vi "Periodic Tasks.vi"(8 "error in":errorcluster) -> ()   [LabVIEW 2014]
doc: "This VI runs in parallel to other tasks. It can contain as many user-defined periodic loops as you need. These can carry out PID or other sorts of timed response."
uses:
  <vilib>/Rock Robotics/SystemInterfaces/Utilities/FPGA_UtilitiesLED Source.ctl
  <vilib>/Rock Robotics/SystemInterfaces/Utilities/FPGA_UtilitiesLED State.ctl
  <vilib>/Rock Robotics/WPI/Joystick/WPI_JoystickGetSetRefNum.vi
  <vilib>/Rock Robotics/WPI/RobotDrive/WPI_RobotDriveGetSetRefNum.vi
  <vilib>/Rock Robotics/Network Tables/SD Write Number.vi
  <vilib>/Rock Robotics/Network Tables/SD Write Boolean.vi
  Global 1.vi
  Robot Global Data.vi
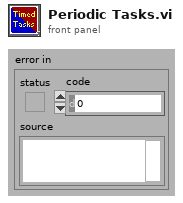
[diagram p1: front panel]
types:
  T1 = typedef "WPI_JoystickDevRef.ctl" = cluster{"Device":T2}
  T2 = typedef "WPI_JoystickDeviceEnum.ctl" = enum16{"USB 0", "USB 1", "USB 2", "USB 3", "USB 4", "USB 5"}
  T3 = typedef "WPI_RobotDriveDevRef.ctl" = cluster{"DevStatus":errorcluster, "Motors[]":T4[], "Square Inputs":bool, "Max Output":dbl}
  T4 = typedef "WPI_MotorControlDeviceRef.ctl" = cluster{"DeviceStatus":errorcluster, "Type":enum16{"PWM", "CAN"}, "PWM":cluster{"Digital Module":T5, "PWM Channel":T6, "DeadBand":T7}, "CAN":cluster{"Device Number":u8, "Control Mode":T8, "Semaphore":T9, "Max Vout":dbl}, "Invert":bool, "TransformRef":T10, "InvTransformRef":T10}
  T5 = typedef "FPGA_TypedefDigitalModule.ctl" = enum16{"Digital Module 1", "Digital Module 2"}
  T6 = typedef "FPGA_DIOPWMChannel.ctl" = enum8{"PWM 1", "PWM 2", "PWM 3", "PWM 4", "PWM 5", "PWM 6", "PWM 7", "PWM 8", "PWM 9", "PWM 10", "Invalid"}
  T7 = typedef "WPI_PWMDeadband.ctl" = cluster{"Name":string, "maxPositivePwm":i32, "minPositivePwm":i32, "centerPwm":i32, "maxNegativePwm":i32, "minNegativePwm":i32, "angularRange":u16}
  T8 = typedef "WPI_CANJaguar_ControlMode.ctl" = enum8{"Percent VBus", "Current", "Speed", "Position", "Voltage"}
  T9 = typedef "Semaphore RefNum" = refnum<k1>
  T10 = typedef "WPI_PWMTransform_ConPane.ctl" = refnum<vi>
  T11 = cluster{"JoystickDevRef":T1, "RobotDriveDevRef":T3}
  T12 = typedef "WPI_EncoderDevRef.ctl" = cluster{"DevStatus":errorcluster, "EncoderIndex":T13, "CounterIndex":T14, "DistancePerCount":dbl, "Decoding Type":T15}
  T13 = typedef "FPGA_EncoderIdx.ctl" = enum8{"Enc 0", "Enc 1", "Enc 2", "Enc 3", "Invalid"}
  T14 = typedef "FPGA_CounterCtrSystemIndex.ctl" = enum8{"Ctr 0", "Ctr 1", "Ctr 2", "Ctr 3", "Ctr 4", "Ctr 5", "Ctr 6", "Ctr 7", "Invalid"}
  T15 = typedef "WPI_EncoderType.ctl" = enum16{"1x", "2x", "4x"}
  T16 = typedef "FPGA_UtilitiesLED State.ctl" = enum16{"Off", "On", "Toggle"}
  T17 = typedef "FPGA_UtilitiesLED Source.ctl" = enum16{"User LED", "FPGA LED"}
  T18 = typedef "WPI_CompressorDevRef.ctl" = cluster{"DevStatus":errorcluster, "DigitalInputDevRef":T19, "RelayDevRef":T21}
  T19 = typedef "WPI_DigitalInputDevRef.ctl" = cluster{"DevStatus":errorcluster, "DIO Channel":T20, "Digital Module":T5}
  T20 = typedef "FPGA_DIOChannel.ctl" = enum8{"DIO 1", "DIO 2", "DIO 3", "DIO 4", "DIO 5", "DIO 6", "DIO 7", "DIO 8", "DIO 9", "DIO 10", "DIO 11", "DIO 12", "DIO 13", "DIO 14", "Invalid"}
  T21 = typedef "WPI_RelayDevRef.ctl" = cluster{"DevStatus":errorcluster, "Relay Channel":T22, "Digital Module":T5, "Relay Direction":T23}
  T22 = typedef "FPGA_DIORelayChannel.ctl" = enum8{"Relay 1", "Relay 2", "Relay 3", "Relay 4", "Relay 5", "Relay 6", "Relay 7", "Relay 8", "Invalid"}
  T23 = typedef "WPI_RelayDirection.ctl" = enum16{"Both directions", "Forward only", "Reverse only"}
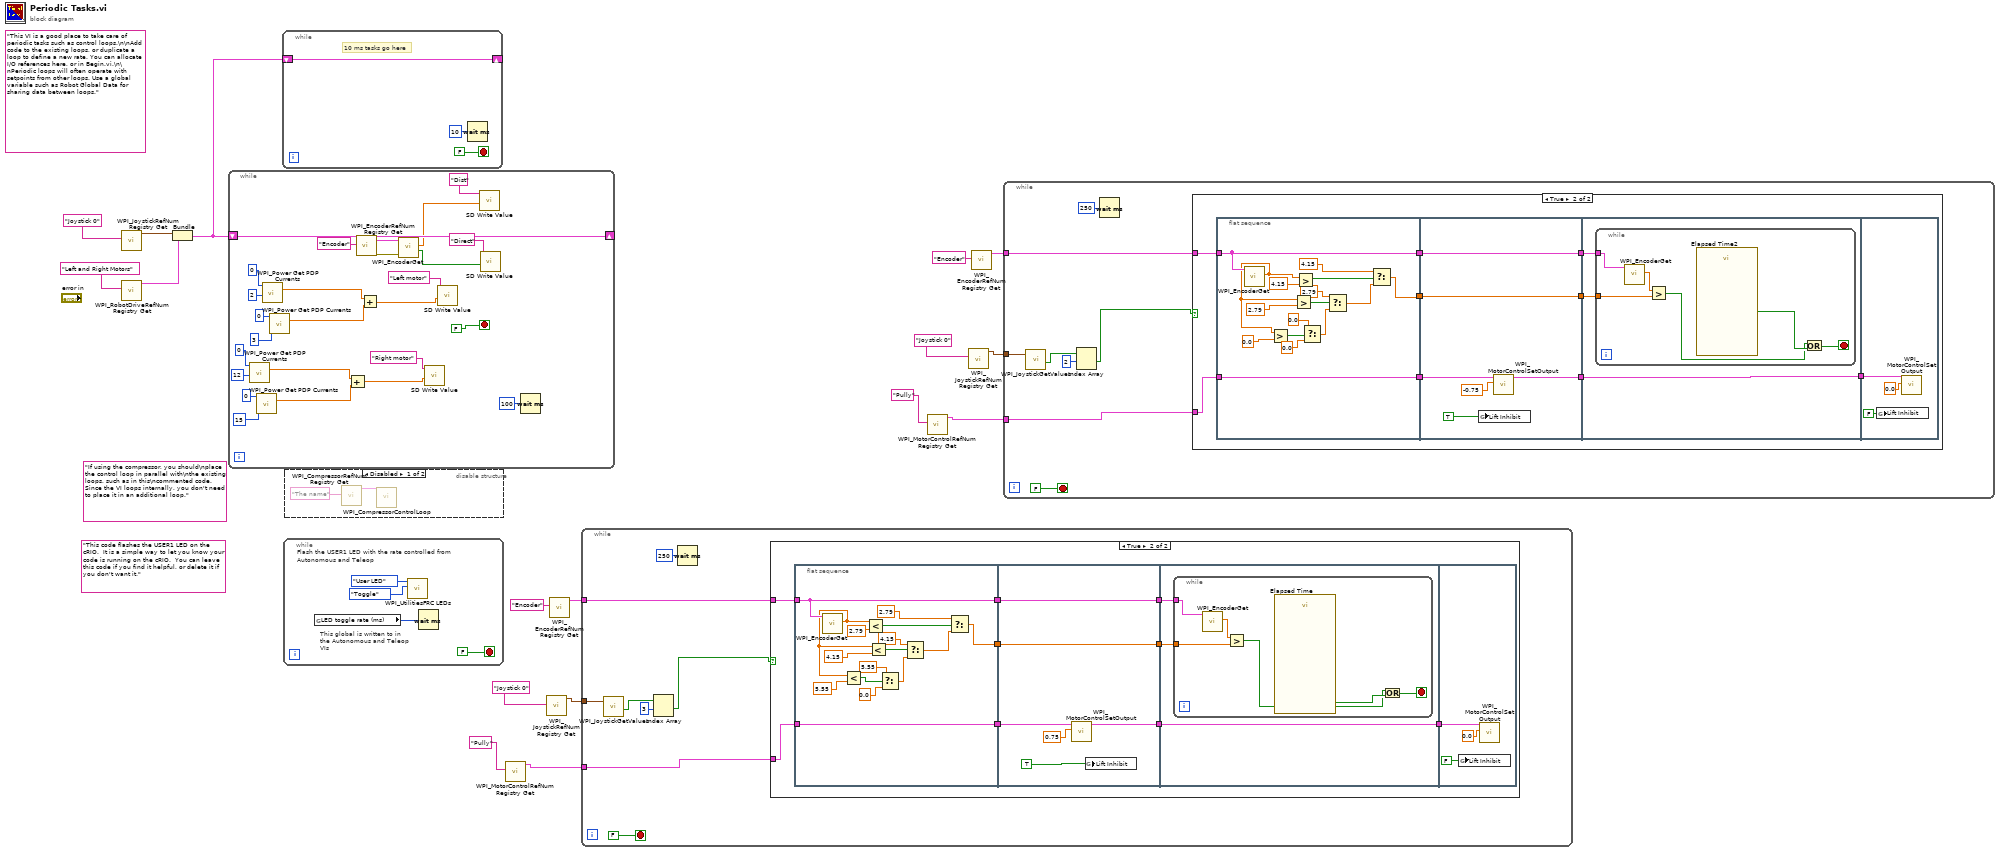
[diagram p0: block diagram]
diagram:
  (unwired) "If using the compressor, you should\nplace the control loop in parallel with\nthe existing loops, such as in this\ncommented code. Since the VI loops internally, you don't need to place it in an additional loop."
  (unwired) "This code flashes the USER1 LED on the cRIO.  It is a simple way to let you know your code is running on the cRIO.  You can leave this code if you find it helpful, or delete it if you don't want it."
  (unwired) "This VI is a good place to take care of periodic tasks such as control loops.\n\nAdd code to the existing loops, or duplicate a loop to define a new rate. You can allocate I/O references here, or in Begin.vi.\n\nPeriodic loops will often operate with setpoints from other loops. Use a global variable such as Robot Global Data for sharing data between loops."
  n1 = call <vilib>:"WPI_JoystickRefNum Registry Get.vi"("refnum name"="Joystick 0") -> ("JoystickDevRef"=w15:T1)  [unwired: 1 in, 9 out]
  n2 = call <vilib>:"WPI_RobotDriveRefNum Registry Get.vi"("refnum name"="Left and Right Motors") -> ("RobotDriveDevRef"=w14:T3)  [unwired: 1 in, 9 out]
  n3 = Bundle("JoystickDevRef"=w15, "RobotDriveDevRef"=w14) -> (w13:T11)  [unwired: 1 out]
  n4 = while {
    shift-right: [w43] -> _
    shift-left: w13 -> [w43]
    stop <- FALSE stop-if-true
    n5 = call <vilib>:"WPI_Power Get PDP Currents.vi"("Power Distribution Panel (0)"=u8 0, "PDP Channel"=12) -> ("current (A)"=w29:dbl)  [unwired: 11 in, 2 out]
    n6 = call <vilib>:"WPI_Power Get PDP Currents.vi"("Power Distribution Panel (0)"=u8 0, "PDP Channel"=15) -> ("current (A)"=w28:dbl)  [unwired: 11 in, 2 out]
    n7 = call <vilib>:"WPI_Power Get PDP Currents.vi"("Power Distribution Panel (0)"=u8 0, "PDP Channel"=2) -> ("current (A)"=w37:dbl)  [unwired: 11 in, 2 out]
    n8 = call <vilib>:"WPI_Power Get PDP Currents.vi"("Power Distribution Panel (0)"=u8 0, "PDP Channel"=3) -> ("current (A)"=w36:dbl)  [unwired: 11 in, 2 out]
    n9 = Add(x=w29, y=w28) -> (x+y=w27:dbl)
    n10 = call <vilib>:"WPI_EncoderRefNum Registry Get.vi"("refnum name"="Encoder") -> ("error out"=w21:errorcluster, "EncoderDevRef"=w20:T12)  [unwired: 9 in]
    n11 = Add(x=w37, y=w36) -> (x+y=w35:dbl)
    n12 = call <vilib>:"WPI_EncoderGet.vi"("error in (no error)"=w21, "EncoderDevRef"=w20) -> ("Direction"=w24:bool, "Distance"=w22:dbl)  [unwired: 4 in, 4 out]
    n13 = call-poly <vilib>:"SD Write Value.vi"("Numeric"=w27, "Name"="Right motor") -> ()  [unwired: 8 in, 2 out]
    n14 = call-poly <vilib>:"SD Write Value.vi"("Numeric"=w35, "Name"="Left motor") -> ()  [unwired: 8 in, 2 out]
    n15 = call-poly <vilib>:"SD Write Value.vi"("Numeric"=w22, "Name"="Dist") -> ()  [unwired: 8 in, 2 out]
    n16 = call-poly <vilib>:"SD Write Value.vi"("Boolean"=w24, "Name"="Direct") -> ()  [unwired: 8 in, 2 out]
    n17 = Wait (ms)(milliseconds to wait=u32 100) -> ()  [unwired: 1 out]
  }
  n18 = while {
    shift-right: [w44] -> _
    shift-left: w13 -> [w44]
    stop <- FALSE stop-if-true
    # "10 ms tasks go here"
    n19 = Wait (ms)(milliseconds to wait=u32 10) -> ()  [unwired: 1 out]
  }
  n20 = while {
    stop <- FALSE stop-if-true
    # "This global is written to in the Autonomous and Teleop VIs"
    # "Flash the USER1 LED with the rate controlled from Autonomous and Teleop"
    n21 = global read "Robot Global Data.vi" "LED toggle rate (ms)"() -> (w47:u32)
    n22 = call <vilib>:"WPI_UtilitiesFRC LEDs.vi"("State"=FPGA_UtilitiesLED_State."Toggle", "LED Type"=FPGA_UtilitiesLED_Source."User LED") -> ()  [unwired: 1 in, 9 out]
    n23 = Wait (ms)(milliseconds to wait=w47) -> ()  [unwired: 1 out]
  }
  n24 = disable-structure shown="Disabled" {
    frame Disabled {
      n25 = call <vilib>:"WPI_CompressorRefNum Registry Get.vi"("refnum name"="The name") -> ("CompressorDevRef"=w52:T18)  [unwired: 9 in, 1 out]
      n26 = call <vilib>:"WPI_CompressorControlLoop.vi"("CompressorDevRef"=w52) -> ()  [unwired: 11 in]
    }
    frame Enabled {
    }
  }
  n27 = call <vilib>:"WPI_MotorControlRefNum Registry Get.vi"("refnum name"="Pully") -> ("MotorControlDevRef"=w11:T4)  [unwired: 9 in, 1 out]
  n28 = call <vilib>:"WPI_JoystickRefNum Registry Get.vi"("refnum name"="Joystick 0") -> ("JoystickDevRef"=w9:T1)  [unwired: 9 in, 1 out]
  n29 = call <vilib>:"WPI_EncoderRefNum Registry Get.vi"("refnum name"="Encoder") -> ("EncoderDevRef"=w8:T12)  [unwired: 9 in, 1 out]
  n30 = while {
    tunnel: w11 -> [w59]
    tunnel: w9 -> [w57]
    tunnel: w8 -> [w54]
    stop <- FALSE stop-if-true
    n31 = call <vilib>:"WPI_JoystickGetValues.vi"("JoystickDevRef"=w57) -> ("Buttons"=w56:bool[])  [unwired: 6 in, 4 out]
    n32 = Index Array(array=w56, index #1=3 ("index")) -> (element #1=w53:bool)  [unwired: 1 in, 1 out]
    n33 = Wait (ms)(milliseconds to wait=u32 250) -> ()  [unwired: 1 out]
    n34 = case shown="True" w53 {
      tunnel: w59 -> [_ w67]
      tunnel: w54 -> [_ w66]
      frame False {
      }
      frame True {
        n35 = flat-sequence {
          tunnel: w66 -> [w84]
          tunnel: w67 -> [w85]
          tunnel: [w85] -> w64
          tunnel: [w84] -> w63
          tunnel: [w70] -> w61
          tunnel: [w90] -> w69
          tunnel: [w88] -> w65
          tunnel: w64 -> [w91]
          tunnel: w63 -> [w88]
          tunnel: [w87] -> w62
          tunnel: w61 -> [w87]
          tunnel: w69 -> [w94]
          tunnel: [w94] -> w68
          tunnel: w65 -> [w93]
          tunnel: w62 -> [w92]
          tunnel: w68 -> [w103]
          frame #0 {
            n36 = call <vilib>:"WPI_EncoderGet.vi"("EncoderDevRef"=w84) -> ("Distance"=w79:dbl)  [unwired: 5 in, 5 out]
            n37 = Less?(x=w79, y=5.55) -> (x < y?=w74:bool)
            n38 = Less?(x=w79, y=2.79) -> (x < y?=w82:bool)
            n39 = Less?(x=w79, y=4.15) -> (x < y?=w75:bool)
            n40 = Select(t=5.55, s=w74, f=0.0) -> (s? t:f=w76:dbl)
            n41 = Select(t=4.15, s=w75, f=w76) -> (s? t:f=w77:dbl)
            n42 = Select(t=2.79, s=w82, f=w77) -> (s? t:f=w70:dbl)
          }
          frame #1 {
            n43 = call <vilib>:"WPI_MotorControlSetOutput.vi"("Output"=0.75, "MotorControlDevRef"=w91) -> ("MotorControlDevRef"=w90:T4)  [unwired: 7 in, 2 out]
            n44 = global write "Global 1.vi" "Lift Inhibit"(TRUE ("Lift Inhibit")) -> ()
          }
          frame #2 {
            n45 = while {
              tunnel: w93 -> [w97]
              tunnel: w92 -> [w95]
              stop <- w99 stop-if-true
              n46 = call <vilib>:"WPI_EncoderGet.vi"("EncoderDevRef"=w97) -> ("Distance"=w98:dbl)  [unwired: 5 in, 5 out]
              n47 = Greater?(x=w98, y=w95) -> (0:w96:bool)
              n48 = call "Elapsed Time"() -> ("Time has Elapsed"=w100:bool)  [unwired: 12 in, 7 out]
              n49 = Or(x=w96, y=w100) -> (x .or. y?=w99:bool)
            }
          }
          frame #3 {
            n50 = global write "Global 1.vi" "Lift Inhibit"(FALSE ("Lift Inhibit")) -> ()
            n51 = call <vilib>:"WPI_MotorControlSetOutput.vi"("Output"=0.0, "MotorControlDevRef"=w103) -> ()  [unwired: 7 in, 3 out]
          }
        }
      }
    }
  }
  n52 = call <vilib>:"WPI_MotorControlRefNum Registry Get.vi"("refnum name"="Pully") -> ("MotorControlDevRef"=w5:T4)  [unwired: 9 in, 1 out]
  n53 = call <vilib>:"WPI_JoystickRefNum Registry Get.vi"("refnum name"="Joystick 0") -> ("JoystickDevRef"=w3:T1)  [unwired: 9 in, 1 out]
  n54 = call <vilib>:"WPI_EncoderRefNum Registry Get.vi"("refnum name"="Encoder") -> ("EncoderDevRef"=w2:T12)  [unwired: 9 in, 1 out]
  n55 = while {
    tunnel: w5 -> [w110]
    tunnel: w3 -> [w108]
    tunnel: w2 -> [w105]
    stop <- FALSE stop-if-true
    n56 = call <vilib>:"WPI_JoystickGetValues.vi"("JoystickDevRef"=w108) -> ("Buttons"=w107:bool[])  [unwired: 6 in, 4 out]
    n57 = Index Array(array=w107, index #1=2 ("index")) -> (element #1=w104:bool)  [unwired: 1 in, 1 out]
    n58 = Wait (ms)(milliseconds to wait=u32 250) -> ()  [unwired: 1 out]
    n59 = case shown="True" w104 {
      tunnel: w110 -> [_ w118]
      tunnel: w105 -> [_ w117]
      frame False {
      }
      frame True {
        n60 = flat-sequence {
          tunnel: w117 -> [w135]
          tunnel: w118 -> [w136]
          tunnel: [w136] -> w115
          tunnel: [w135] -> w114
          tunnel: [w128] -> w112
          tunnel: [w141] -> w120
          tunnel: [w139] -> w116
          tunnel: w115 -> [w142]
          tunnel: w114 -> [w139]
          tunnel: [w138] -> w113
          tunnel: w112 -> [w138]
          tunnel: w120 -> [w145]
          tunnel: [w145] -> w119
          tunnel: w116 -> [w144]
          tunnel: w113 -> [w143]
          tunnel: w119 -> [w154]
          frame #0 {
            n61 = call <vilib>:"WPI_EncoderGet.vi"("EncoderDevRef"=w135) -> ("Distance"=w122:dbl)  [unwired: 5 in, 5 out]
            n62 = Greater?(x=w122, y=0.0) -> (0:w126:bool)
            n63 = Greater?(x=w122, y=2.79) -> (0:w125:bool)
            n64 = Greater?(x=w122, y=4.15) -> (0:w123:bool)
            n65 = Select(t=0.0, s=w126, f=0.0) -> (s? t:f=w132:dbl)
            n66 = Select(t=2.79, s=w125, f=w132) -> (s? t:f=w133:dbl)
            n67 = Select(t=4.15, s=w123, f=w133) -> (s? t:f=w128:dbl)
          }
          frame #1 {
            n68 = global write "Global 1.vi" "Lift Inhibit"(TRUE ("Lift Inhibit")) -> ()
            n69 = call <vilib>:"WPI_MotorControlSetOutput.vi"("Output"=-0.75, "MotorControlDevRef"=w142) -> ("MotorControlDevRef"=w141:T4)  [unwired: 7 in, 2 out]
          }
          frame #2 {
            n70 = while {
              tunnel: w144 -> [w148]
              tunnel: w143 -> [w146]
              stop <- w150 stop-if-true
              n71 = call <vilib>:"WPI_EncoderGet.vi"("EncoderDevRef"=w148) -> ("Distance"=w149:dbl)  [unwired: 5 in, 5 out]
              n72 = Greater?(x=w149, y=w146) -> (0:w147:bool)
              n73 = call "Elapsed Time2"() -> ("Time has Elapsed"=w151:bool)  [unwired: 12 in, 7 out]
              n74 = Or(x=w147, y=w151) -> (x .or. y?=w150:bool)
            }
          }
          frame #3 {
            n75 = global write "Global 1.vi" "Lift Inhibit"(FALSE ("Lift Inhibit")) -> ()
            n76 = call <vilib>:"WPI_MotorControlSetOutput.vi"("Output"=0.0, "MotorControlDevRef"=w154) -> ()  [unwired: 7 in, 3 out]
          }
        }
      }
    }
  }
